vi "Send illumination arm.vi"(8 "error in (no error)":errorcluster, 11 "Tomo in":refnum<class "Tomo.lvclass">) -> (0 "error out":errorcluster, 3 "Tomo out":refnum<class "Tomo.lvclass">)   [LabVIEW 2012, in "Tomo.lvclass"]
uses:
  Tomo.lvclass
  <vilib>/Distrio/Murmex/Murmex/update_cluster.ctl
  <vilib>/Distrio/Murmex/Murmex/Murmex.lvclass
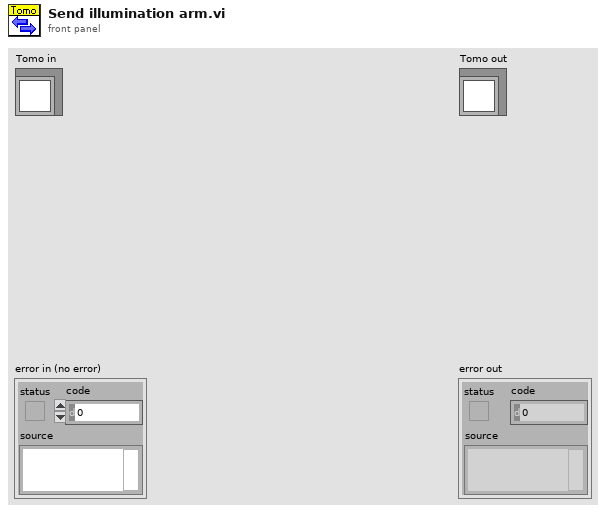
[diagram p1: front panel]
types:
  T1 = typedef "Murmex.lvlib/Murmex.lvclass/update_cluster.ctl" = cluster{"target ID":string, "key chains":string[], "values":variant[]}
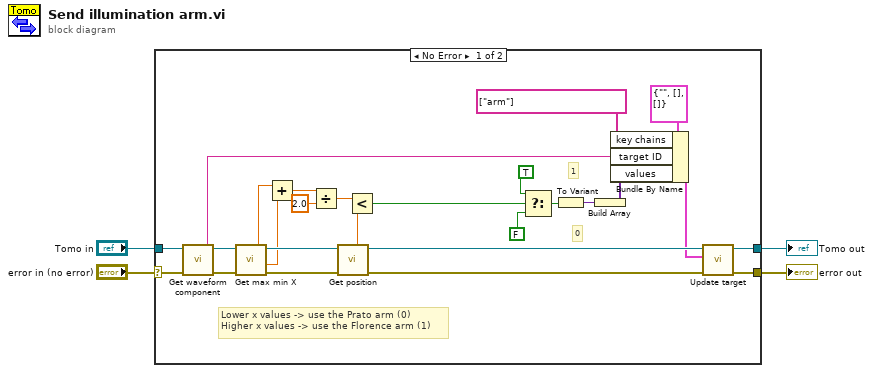
[diagram p0: block diagram]
diagram:
  n1 = case shown="No Error" "error in (no error)" {
    selector: "error in (no error)" -> [w30 w32]
    tunnel: [w23 w32] -> w3
    tunnel: [w21 w31] -> w1
    tunnel: "Tomo in" -> [w25 w31]
    frame No Error {
      # "0"
      # "1"
      # "Lower x values -> use the Prato arm (0)\nHigher x values -> use the Florence arm (1)"
      n2 = call-dynamic "Get waveform component.vi"("error in (no error)"=w30, "Tomo in"=w25) -> ("error out"=w26:errorcluster, "waveform component"=w18:string, "Tomo out"=w24:refnum<class "Tomo.lvclass">)  [unwired: 7 in]
      n3 = call-dynamic "Get max min X.vi"("error in (no error)"=w26, "Tomo in"=w24) -> ("error out"=w29:errorcluster, "X max"=w14:dbl[unit], "X min"=w15:dbl[unit], "Tomo out"=w27:refnum<class "Tomo.lvclass">)  [unwired: 6 in]
      n4 = Add(x=w15, y=w14) -> (x+y=w16:dbl[unit])
      n5 = Divide(x=w16, y=2.0) -> (x/y=w12:dbl[unit])
      n6 = call-dynamic "Get position.vi"("error in (no error)"=w29, "Tomo in"=w27) -> ("error out"=w28:errorcluster, "Tomo out"=w22:refnum<class "Tomo.lvclass">, "X position"=w11:dbl[unit])  [unwired: 4 in, 3 out]
      n7 = Less?(x=w12, y=w11) -> (x < y?=w10:bool)
      n8 = Select(t=TRUE, s=w10, f=FALSE) -> (s? t:f=w9:bool)
      n9 = To Variant(anything=w9) -> (Variant=w8:variant)
      n10 = Build Array(w8) -> (w7:variant[])
      n11 = Bundle By Name(cluster=T1 {"target ID"="", "key chains"=[], "values"=[]} ("update cluster"), "key chains"=string[] ["arm"], "target ID"=w18, "values"=w7) -> (w17:T1)
      n12 = call <vilib>:"Update target.vi"("error in (no error)"=w28, "update cluster"=w17, "MurmexBase in"=w22) -> ("error out"=w23:errorcluster, "MurmexBase out"=w21:refnum<class "Tomo.lvclass">)  [unwired: 7 in]
    }
    frame Error {
    }
  }
  "error out" <- w3
  "Tomo out" <- w1
